vi "Advanced Trigger Detector.vi"(0 "data in":dbl[](array[numeric]), 1 "reset? (F)":bool, 5 "triggers definition":T2(array[cluster]), 9 "data timestamp":timestamp, 11 "error in (no error)":errorcluster) -> (4 "triggers":T1(array[cluster]), 6 "actual trigger state":bool[](array[boolean]), 15 "error out":errorcluster)   [LabVIEW 2012, in "NI_EP_Power Quality.lvlib"]
doc: "Combines multiple trigger conditions using boolean operators and detects whether the combined trigger occurs. You can specify multiple combined triggers."
uses:
  <vilib>/addons/Electrical Power/PQ/NI_EP_Power Quality.lvlib
  <vilib>/addons/Electrical Power/PQ/Triggers/subVIs/ep_Trigger Definition.ctl
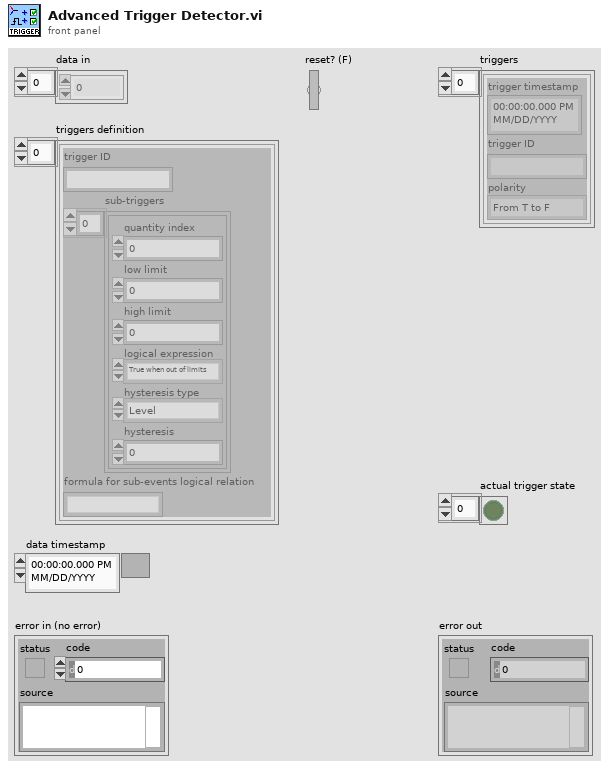
[diagram p1: front panel]
types:
  T1 = cluster{"trigger timestamp":timestamp, "trigger ID":string, "polarity":enum16{"From T to F", "From F to T"}}[]
  T2 = cluster{"trigger ID":string, "sub-triggers":cluster{"quantity index":u32, "low limit":dbl, "high limit":dbl, "logical expression":enum16{"True when out of limits", "True when in limits"}, "hysteresis type":enum16{"Level", "Time"}, "hysteresis":dbl}[], "formula for sub-events logical relation ":string}[]
  T3 = cluster{"data time stamp":timestamp, "trigger unique id":string, "f":enum16{"From T to F", "From F to T"}}[]
  T4 = typedef "NI_EP_Power Quality.lvlib/ep_Trigger Definition.ctl" = cluster{"trigger ID":string, "low limit":dbl, "high limit":dbl, "direction":enum16{"Out of limits", "Back to limits", "Both"}, "hysteresis type":enum16{"Level", "Time"}, "hysteresis":dbl}
  T5 = cluster{T4[], i8[], cluster{"Lo in progr.":bool, "Hi in progr.":bool, "Lo trig. time":timestamp, "Hi trig. time":timestamp}[], "result":bool}[]
  T6 = cluster{"quantity index":u32, "low limit":dbl, "high limit":dbl, "logical expression":enum16{"True when out of limits", "True when in limits"}, "hysteresis type":enum16{"Level", "Time"}, "hysteresis":dbl}[]
  T7 = cluster{T4[], i8[], cluster{"Lo in progr.":bool, "Hi in progr.":bool, "Lo trig. time":timestamp, "Hi trig. time":timestamp}[], "result":bool}
  T8 = cluster{"Lo in progr.":bool, "Hi in progr.":bool, "Lo trig. time":timestamp, "Hi trig. time":timestamp}[]
  T9 = cluster{"Lo in progr.":bool, "Lo in progr.":bool, "data timestamp":timestamp, "data timestamp":timestamp}
  T10 = enum16{"True when out of limits", "True when in limits"}
  T11 = cluster{"Lo in progr.":bool, "Hi in progr.":bool, "Lo trig. time":timestamp, "Hi trig. time":timestamp}
  T12 = cluster{"data timestamp":timestamp, "trigger ID":string, "f":enum16{"From T to F", "From F to T"}}
  T13 = cluster{"data timestamp":timestamp, "trigger ID":string, "f":enum16{"From T to F", "From F to T"}}[]
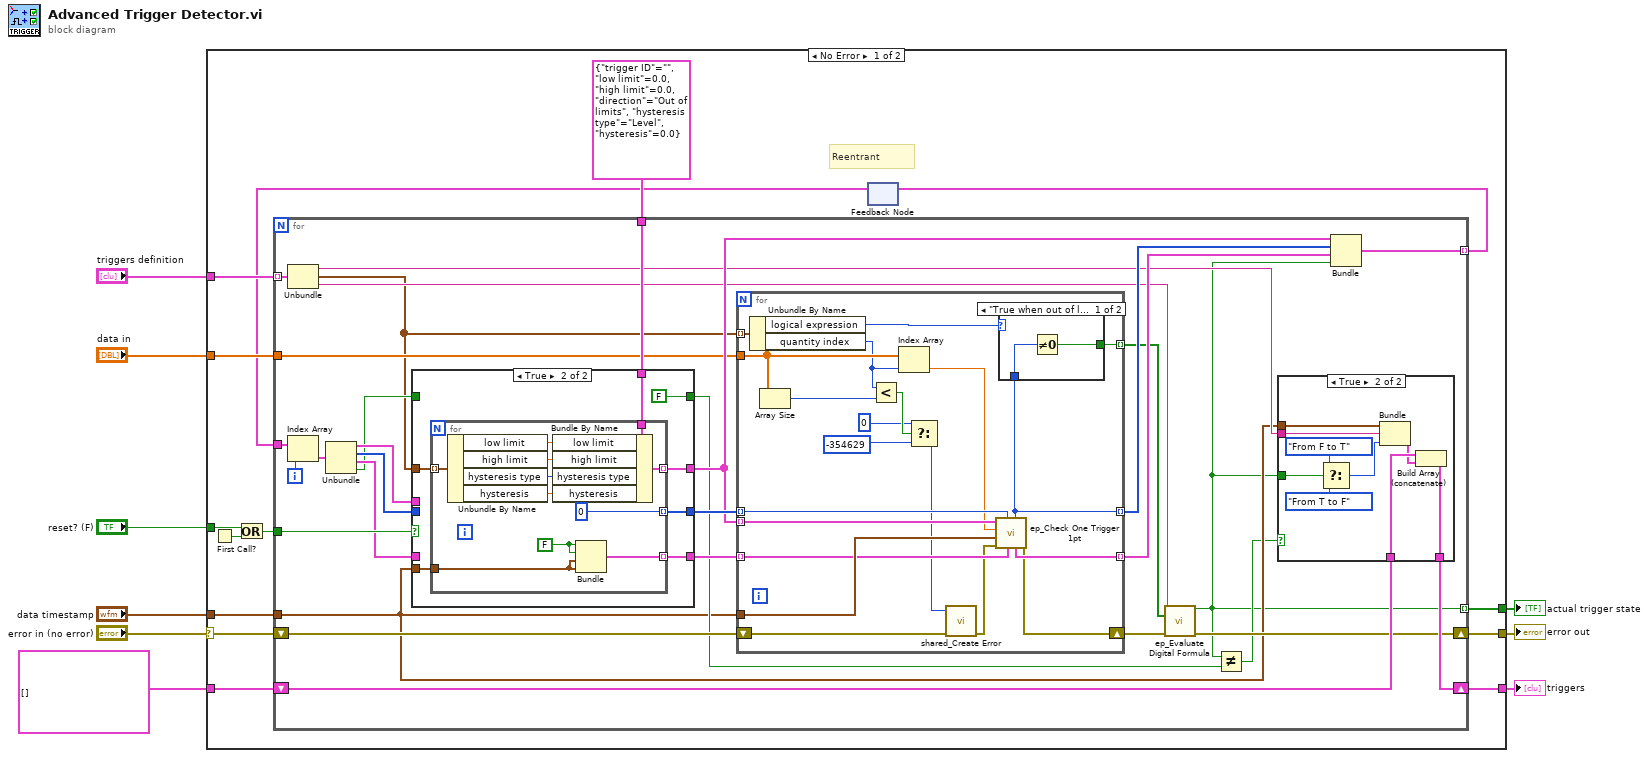
[diagram p0: block diagram]
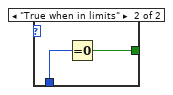
[diagram p4: hidden frame]
diagram:
  n1 = case shown="No Error" "error in (no error)" {
    selector: "error in (no error)" -> [w17 w111]
    tunnel: "data in" -> [w23 _]
    tunnel: "reset? (F)" -> [w21 _]
    tunnel: "data timestamp" -> [w18 _]
    tunnel: [w16 w111] -> w9
    tunnel: "triggers definition" -> [w15 _]
    tunnel: T3 [] -> [w13 w110]
    tunnel: [w12 w110] -> w2
    tunnel: [w10 _] -> w1
    frame No Error {
      # "Reentrant"
      n2 = First Call?() -> (First Call?: T/F=w22:bool)
      n3 = Or(x=w21, y=w22) -> (x .or. y?=w20:bool)
      n4 = feedback #1() -> (w11:T5)  [unwired: 1 in]
      n5 = for {
        tunnel: w23 -> [w41]
        tunnel: w20 -> [w53]
        tunnel: T4 {"trigger ID"="", "low limit"=0.0, "high limit"=0.0, "direction"=enum."Out of limits", "hysteresis type"=enum."Level", "hysteresis"=0.0} ("trigger definition") -> [w52]
        tunnel: w18 -> [w27]
        shift-right: [w31] -> w16
        shift-left: w17 -> [w39]
        tunnel: w15 -> [w42] mode=indexing
        tunnel: [w46] -> w14 mode=indexing
        shift-right: [w34] -> w12
        shift-left: w13 -> [w35]
        tunnel: w11 -> [w30]
        tunnel: [w24] -> w10 mode=indexing
        i -> [w29]
        n6 = Unbundle(w42) -> ("trigger ID"=w36:string, "sub-triggers"=w25:T6, "formula for sub-events logical relation"=w33:string)
        n7 = Index Array(array=w30, index=w29) -> (element=w28:T7)
        n8 = Unbundle(w28) -> (w43:T4[], w45:i8[], w44:T8, "result"=w40:bool)
        n9 = case shown="True" w53 {
          tunnel: w25 -> [_ w74]
          tunnel: [w65 w73] -> w49
          tunnel: w52 -> [_ w72]
          tunnel: [w67 w71] -> w51
          tunnel: [w66 w70] -> w50
          tunnel: w45 -> [w66 _]
          tunnel: w44 -> [w67 _]
          tunnel: w27 -> [_ w69]
          tunnel: w43 -> [w65 _]
          tunnel: [w64 FALSE] -> w37
          tunnel: w40 -> [w64 _]
          frame False {
          }
          frame True {
            n10 = for {
              tunnel: w74 -> [w83] mode=indexing
              tunnel: [w82] -> w73 mode=indexing
              tunnel: w72 -> [w81]
              tunnel: [w77] -> w71 mode=indexing
              tunnel: [i8 0] -> w70 mode=indexing
              tunnel: w69 -> [w78]
              w79 = FALSE ("Lo in progr.")
              n11 = Unbundle By Name(w83) -> ("low limit"=w76:dbl, "high limit"=w75:dbl, "hysteresis type"=w84:enum16{"Level", "Time"}, "hysteresis"=w85:dbl)
              n12 = Bundle By Name(cluster=w81, "low limit"=w76, "high limit"=w75, "hysteresis type"=w84, "hysteresis"=w85) -> (w82:T4)
              n13 = Bundle("Lo in progr."=w79, "Lo in progr."=w79, "data timestamp"=w78, "data timestamp"=w78) -> (w77:T9)  [unwired: 1 in]
            }
          }
        }
        n14 = for {
          tunnel: w27 -> [w103]
          tunnel: w25 -> [w101] mode=indexing
          tunnel: w41 -> [w98]
          tunnel: w51 -> [w100] mode=indexing
          tunnel: w50 -> [w104] mode=indexing
          tunnel: [w93] -> w48 mode=indexing
          tunnel: [w102] -> w47 mode=indexing
          tunnel: w49 -> [w105] mode=indexing
          shift-right: [w99] -> w32
          shift-left: w39 -> [w88]
          tunnel: [w92] -> w38 mode=indexing
          n15 = Unbundle By Name(w101) -> ("logical expression"=w94:T10, "quantity index"=w91:u32)
          n16 = Array Size(array=w98) -> (size(s)=w97:i32)
          n17 = Less?(x=w91, y=w97) -> (x < y?=w96:bool)
          n18 = Index Array(array=w98, index=w91) -> (element=w95:dbl)
          n19 = Select(t=0 ("error code (0)"), s=w96, f=-354629 ("error code (0)")) -> (s? t:f=w86:i32)
          n20 = call <vilib>:"shared_Create Error.vi"("error in (no error)"=w88, "error code (0)"=w86) -> ("error out"=w87:errorcluster)  [unwired: 9 in]
          n21 = call <vilib>:"ep_Check One Trigger 1pt.vi"("trig. local in"=w100, "prev. state in"=w104, "error in (no error)"=w87, "data time stamp"=w103, "value in"=w95, "trigger definition"=w105) -> ("error out"=w99:errorcluster, "trig. local out"=w102:T11, "state out"=w93:i8)  [unwired: 2 in, 1 out]
          n22 = case shown="\"True when out of limits\", Default" w94 {
            tunnel: w93 -> [w107 w109]
            tunnel: [w106 w108] -> w92
            frame "True when out of limits", Default {
              n23 = Not Equal To 0?(x=w107) -> (x != 0?=w106:bool)
            }
            frame "True when in limits" {
              n24 = Equal To 0?(x=w109) -> (x = 0?=w108:bool)
            }
          }
        }
        n25 = call <vilib>:"ep_Evaluate Digital Formula.vi"("digital formula"=w33, "digital variables"=w38, "error in (no error)"=w32) -> ("result"=w24:bool, "error out"=w31:errorcluster)  [unwired: 11 in]
        n26 = Not Equal?(x=w24, y=w37) -> (x != y?=w26:bool)
        n27 = case shown="True" w26 {
          tunnel: w24 -> [_ w63]
          tunnel: w36 -> [_ w59]
          tunnel: w27 -> [_ w58]
          tunnel: w35 -> [w54 w57]
          tunnel: [w54 w55] -> w34
          frame False {
          }
          frame True {
            n28 = Select(t=enum16{"From T to F", "From F to T"}."From F to T" ("polarity"), s=w63, f=enum16{"From T to F", "From F to T"}."From T to F") -> (s? t:f=w60:enum16{"From T to F", "From F to T"})
            n29 = Bundle("data timestamp"=w58, "trigger ID"=w59, "f"=w60) -> (w56:T12)  [unwired: 1 in]
            n30 = Build Array (concatenate)(w57, w56) -> (w55:T13)
          }
        }
        n31 = Bundle(w49, w48, w47, "result"=w24) -> (w46:T7)  [unwired: 1 in]
      }
      n32 = feedback-in #1(w14) -> ()
    }
    frame Error {
    }
  }
  "error out" <- w9
  "triggers" <- w2
  "actual trigger state" <- w1
